vi "Read States Data.vi"(8 "error in (no error)":errorcluster, 11 "Debugger in":refnum<class "Debugger.lvclass">) -> (0 "error out":errorcluster, 2 "State Map":map{string, string}(c390), 3 "Debugger in 2":refnum<class "Debugger.lvclass">)   [LabVIEW 2020, in "Debugger.lvclass"]
uses:
  Debugger.lvclass
  State Analyzer/Debug State Analyzer.lvclass/Debug State Analyzer.ctl
  Debugger.lvclass/Debugger.ctl
  State Analyzer/Debug State Analyzer.lvclass
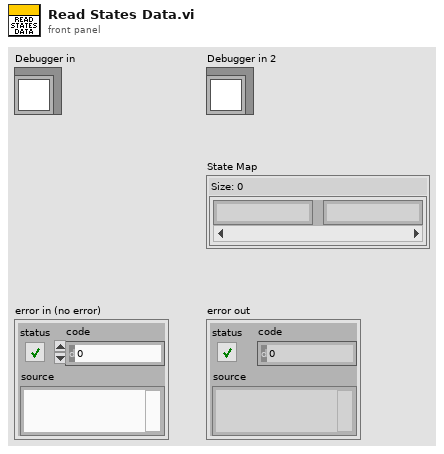
[diagram p1: front panel]
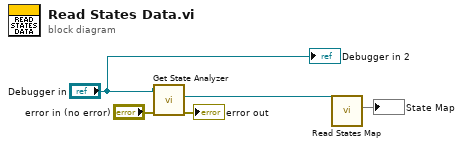
[diagram p0: block diagram]
diagram:
  n1 = call "Get State Analyzer.vi"("error in (no error)"="error in (no error)", "Debugger in"="Debugger in") -> ("error out"=→"error out":errorcluster, "Log"=w3:refnum<class "Debug State Analyzer.lvclass">)  [unwired: 7 in, 1 out]
  n2 = call "Read States Map.vi"("Debug State Analyzer in"=w3) -> ("State Map"=→"State Map":map{string, string})  [unwired: 9 in, 1 out]
  "Debugger in 2" <- "Debugger in"
